vi "crc-8vi.vi"() -> ()   [LabVIEW 2020]
uses:
  CRC SubVIs/Wrappers/CRC-8-CCITT.vi
panel:
  out "CRC-8-CCITT":u8 format="%.0x"
  in  "String":string="this is a test string"
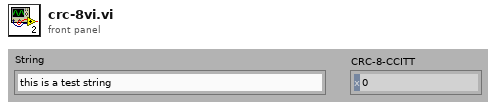
[diagram p1: front panel]
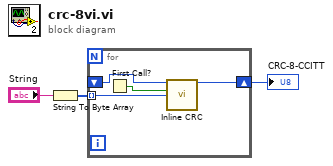
[diagram p0: block diagram]
diagram:
  n1 = String To Byte Array(string="String") -> (unsigned byte array=w3:u8[])
  n2 = for {
    shift-right: [w7] -> w2
    shift-left: _ -> [w6]
    tunnel: w3 -> [w4] mode=indexing
    n3 = First Call?() -> (First Call?: T/F=w5:bool)
    n4 = call-poly "Inline CRC.vi"("CRC In"=w6, "Reset"=w5, "Data"=w4) -> ("CRC"=w7:u8)  [unwired: 11 in, 1 out]
  }
  "CRC-8-CCITT" <- w2
